vi "Run.vi"(8 "error in (no error)":errorcluster, 11 "Simulated VeriStand Engine in":refnum<class "Simulated VeriStand Engine.lvclass">) -> (0 "error out":errorcluster, 3 "Simulated VeriStand Engine out":refnum<class "Simulated VeriStand Engine.lvclass">)   [LabVIEW 2016, in "Simulated VeriStand Engine.lvclass"]
uses:
  Simulated VeriStand Engine.lvclass
  Source/Submodules/Memory/Source/Classes/Pointer/Memory.Pointer.lvclass
  Source/Submodules/Memory/Source/Classes/Internal/Memory.Pointer.Internal.lvclass
  C:/Git/SourceTree/DSF/Source/Submodules/Memory/Source/Classes/Pointer/Memory.Pointer.lvclass
  Source/Submodules/Memory/Source/Classes/Pointer/Memory.Pointer.Write.Safe.0D.U32.vi
  Source/Submodules/Memory/Source/Classes/Pointer/Memory.Pointer.Write.Safe.0D.Bool.vi
  Source/Submodules/Memory/Source/Classes/Pointer/Memory.Pointer.Read.Safe.0D.Bool.vi
  Source/Submodules/Memory/Source/Classes/Pointer/Memory.Pointer.Read.Safe.0D.U32.vi
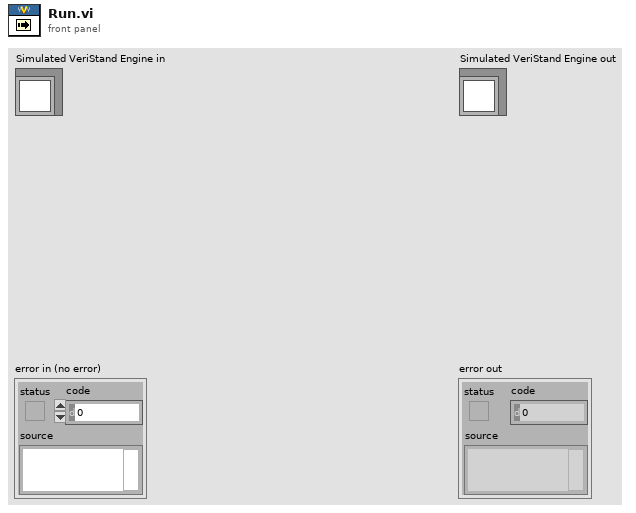
[diagram p1: front panel]
types:
  T1 = typedef "Simulated VeriStand Engine.lvclass/DSF.Engine.Pointers.Status.ctl" = cluster{"actual period":refnum<class "Memory.Pointer.Internal.lvclass">}
  T2 = typedef "Simulated VeriStand Engine.lvclass/DSF.Engine.Pointers.Control.ctl" = cluster{"stop":refnum<class "Memory.Pointer.Internal.lvclass">, "target period":refnum<class "Memory.Pointer.Internal.lvclass">}
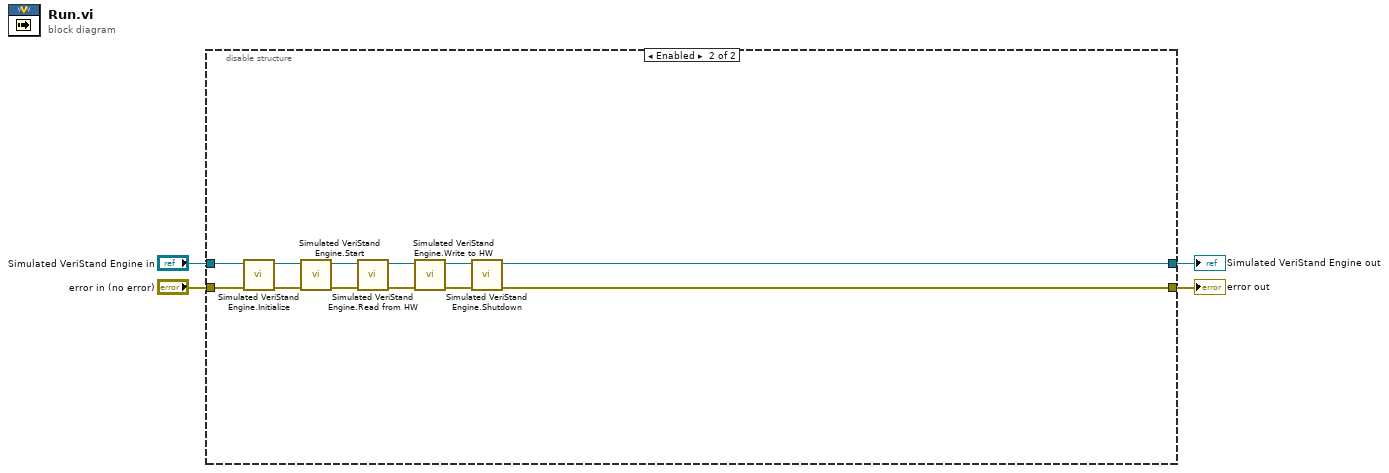
[diagram p0: block diagram]
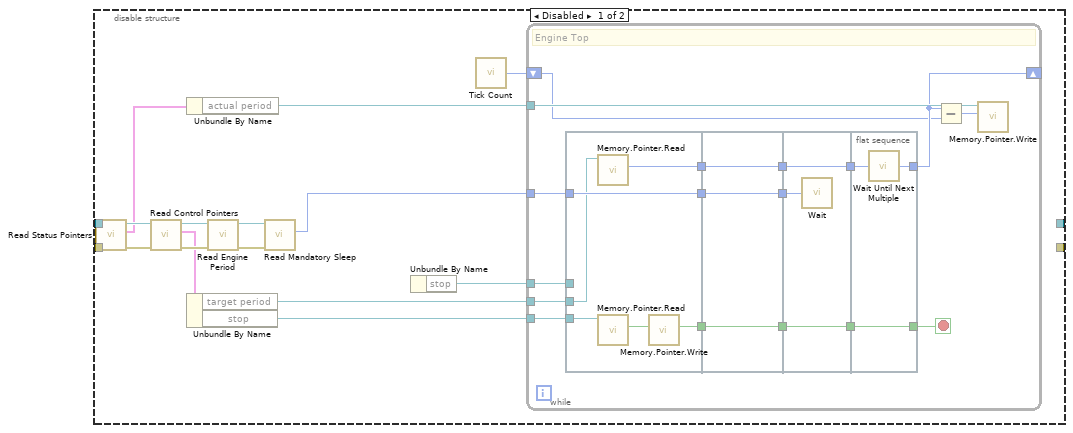
[diagram p2: hidden frame]
diagram:
  n1 = disable-structure shown="Enabled" {
    disable-tunnel: "Simulated VeriStand Engine in" -> [w12 w64]
    disable-tunnel: "error in (no error)" -> [w11 w63]
    disable-tunnel: [_ w54] -> w2
    disable-tunnel: [_ w53] -> w1
    frame Disabled {
      n2 = call "Read Status Pointers.vi"("error in (no error)"=w11, "Simulated VeriStand Engine in"=w12) -> ("error out"=w9:errorcluster, "Status Pointers"=w7:T1, "Simulated VeriStand Engine out"=w10:refnum<class "Simulated VeriStand Engine.lvclass">)  [unwired: 7 in]
      n3 = call "Read Control Pointers.vi"("error in (no error)"=w9, "Simulated VeriStand Engine in"=w10) -> ("error out"=w16:errorcluster, "Control Pointers"=w15:T2, "Simulated VeriStand Engine out"=w17:refnum<class "Simulated VeriStand Engine.lvclass">)  [unwired: 7 in]
      n4 = Unbundle By Name(w7) -> ("actual period"=w6:refnum<class "Memory.Pointer.Internal.lvclass">)
      n5 = Unbundle By Name(w15) -> ("target period"=w8:refnum<class "Memory.Pointer.Internal.lvclass">, "stop"=w14:refnum<class "Memory.Pointer.Internal.lvclass">)
      n6 = call "Read Engine Period.vi"("error in (no error)"=w16, "Simulated VeriStand Engine in"=w17) -> ("error out"=w18:errorcluster, "Simulated VeriStand Engine out"=w19:refnum<class "Simulated VeriStand Engine.lvclass">)  [unwired: 7 in, 1 out]
      n7 = call "Read Mandatory Sleep.vi"("error in (no error)"=w18, "Simulated VeriStand Engine in"=w19) -> ("Mandatory Sleep"=w20:u32)  [unwired: 7 in, 2 out]
      n8 = Unbundle By Name() -> ("stop"=w5:refnum<class "Memory.Pointer.Internal.lvclass">)  [unwired: 1 in]
      n9 = call "Tick Count"() -> ("Tick Count(uSec)"=w13:u32)
      n10 = while {
        tunnel: w20 -> [w37]
        tunnel: w14 -> [w31]
        tunnel: w8 -> [w26]
        shift-right: [w23] -> _
        shift-left: w13 -> [w22]
        tunnel: w6 -> [w24]
        tunnel: w5 -> [w21]
        stop <- w27 stop-if-true
        # "Engine Top"
        n11 = flat-sequence {
          tunnel: w37 -> [w43]
          tunnel: [w43] -> w33
          tunnel: [w41] -> w32
          tunnel: w31 -> [w42]
          tunnel: [w38] -> w30
          tunnel: w26 -> [w40]
          tunnel: w21 -> [_]
          tunnel: [w46] -> w36
          tunnel: [w45] -> w35
          tunnel: w33 -> [w46]
          tunnel: w32 -> [w45]
          tunnel: w30 -> [w44]
          tunnel: [w44] -> w29
          tunnel: w36 -> [w49]
          tunnel: w35 -> [w48]
          tunnel: [w48] -> w34
          tunnel: w29 -> [w47]
          tunnel: [w47] -> w28
          tunnel: w34 -> [w52]
          tunnel: w28 -> [w51]
          tunnel: [w51] -> w27
          tunnel: [w50] -> w23
          frame #0 {
            n12 = call-poly "Memory.Pointer.Read.vi"("pointer in"=w40) -> ("value out"=w41:u32)  [unwired: 7 in, 3 out]
            n13 = call-poly "Memory.Pointer.Read.vi"("pointer in"=w42) -> ("value out"=w39:bool)  [unwired: 7 in, 3 out]
            n14 = call-poly "Memory.Pointer.Write.vi"("value"=w39) -> ("value"=w38:bool)  [unwired: 7 in, 3 out]
          }
          frame #1 {
          }
          frame #2 {
            n15 = call "Wait"("Count(uSec)"=w49) -> ()  [unwired: 1 out]
          }
          frame #3 {
            n16 = call "Wait Until Next Multiple"("Count(uSec)"=w52) -> ("Tick Count(uSec)"=w50:u32)
          }
        }
        n17 = Subtract(x=w23, y=w22) -> (x-y=w25:u32)
        n18 = call-poly "Memory.Pointer.Write.vi"("value"=w25, "pointer in"=w24) -> ()  [unwired: 6 in, 4 out]
      }
    }
    frame Enabled {
      n19 = call-dynamic "Simulated VeriStand Engine.Initialize.vi"("error in (no error)"=w63, "Simulated VeriStand Engine in"=w64) -> ("error out"=w61:errorcluster, "Simulated VeriStand Engine out"=w62:refnum<class "Simulated VeriStand Engine.lvclass">)  [unwired: 8 in]
      n20 = call-dynamic "Simulated VeriStand Engine.Start.vi"("error in (no error)"=w61, "Simulated VeriStand Engine in"=w62) -> ("error out"=w59:errorcluster, "Simulated VeriStand Engine out"=w60:refnum<class "Simulated VeriStand Engine.lvclass">)  [unwired: 8 in]
      n21 = call-dynamic "Simulated VeriStand Engine.Read from HW.vi"("error in (no error)"=w59, "Simulated VeriStand Engine in"=w60) -> ("error out"=w57:errorcluster, "Simulated VeriStand Engine out"=w58:refnum<class "Simulated VeriStand Engine.lvclass">)  [unwired: 8 in]
      n22 = call-dynamic "Simulated VeriStand Engine.Write to HW.vi"("error in (no error)"=w57, "Simulated VeriStand Engine in"=w58) -> ("error out"=w55:errorcluster, "Simulated VeriStand Engine out"=w56:refnum<class "Simulated VeriStand Engine.lvclass">)  [unwired: 8 in]
      n23 = call-dynamic "Simulated VeriStand Engine.Shutdown.vi"("error in (no error)"=w55, "Simulated VeriStand Engine in"=w56) -> ("error out"=w53:errorcluster, "Simulated VeriStand Engine out"=w54:refnum<class "Simulated VeriStand Engine.lvclass">)  [unwired: 8 in]
    }
  }
  "error out" <- w1
  "Simulated VeriStand Engine out" <- w2
